vi "Subvitwmp (SubVI).vi"(11 "Temp in C":dbl) -> (3 "Temp in F":dbl)   [LabVIEW 2019]
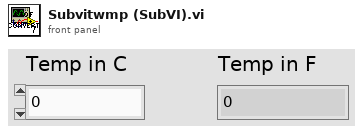
[diagram p1: front panel]
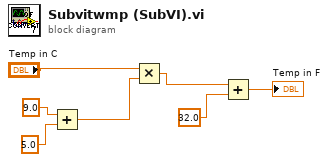
[diagram p0: block diagram]
diagram:
  n1 = Add(x=9.0 ("y"), y=5.0) -> (x+y=w1:dbl)
  n2 = Multiply(x="Temp in C", y=w1) -> (x*y=w3:dbl)
  n3 = Add(x=w3, y=32.0) -> (x+y=→"Temp in F":dbl)
